vi "K2450 Set Volt.vi"(8 "error in (no error)":errorcluster {"code" format="%.0x"}, 10 "Voltage 2450":dbl, 11 "VISA resource name":refnum<visa-resource-name>) -> (0 "error out":errorcluster {"code" format="%.0x"}, 2 "Write ∆ Time [ms]":dbl format="%.4f", 3 "dup VISA Session":refnum<visa-resource-name>)   [LabVIEW 2025]
doc: "Author: Scott Hannahs <sth@magnet.fsu.edu>\n\nThis software is licensed for use under the “MIT License\"\nCopyright (c) 2025 Scott Hannahs, sth@sth@magnet.sthnet.net\n\nPermission is hereby granted, free of charge, to any person obtaining a copy of this software and associated documentation files (the \"Software\"), to deal in the Software without restriction, including without limitation the rights to use, copy, modify, merge, publish, distribute, sublicense, and/or sell copies of the Software, and to permit persons to whom the Software is furnished to do so, subject to the following conditions: The above copyright notice and this permission notice shall be included in all copies or substantial portions of the Software.\n\nTHE SOFTWARE IS PROVIDED \"AS IS\", WITHOUT WARRANTY OF ANY KIND, EXPRESS OR IMPLIED, INCLUDING BUT NOT LIMITED TO THE WARRANTIES OF MERCHANTABILITY, FITNESS FOR A PARTICULAR PURPOSE AND NONINFRINGEMENT. IN NO EVENT SHALL THE AUTHORS OR COPYRIGHT HOLDERS BE LIABLE FOR ANY CLAIM, DAMAGES OR OTHER LIABILITY, WHETHER IN AN ACTION OF CONTRACT, TORT OR OTHERWISE, ARISING FROM, OUT OF OR IN CONNECTION WITH THE SOFTWARE OR THE USE OR OTHER DEALINGS IN THE SOFTWARE."
panel:
  # "Make sure unit is set to source V\nsour:func volt\nAnd turned on\nOUTPut ON"
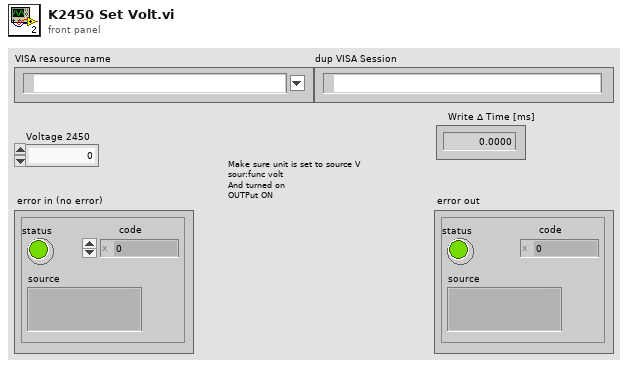
[diagram p1: front panel]
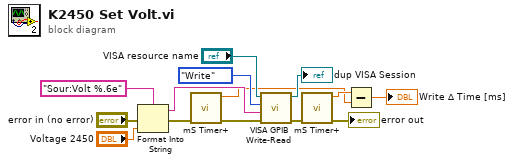
[diagram p0: block diagram]
diagram:
  n1 = Format Into String(format string="Sour:Volt %.6e" ("Command"), error in="error in (no error)", "Voltage 2450") -> (resulting string=w10:string, error out=w5:errorcluster)  [unwired: 1 in]
  n2 = call "mS Timer+.vi"("Error In"=w5) -> ("Error Out"=w4:errorcluster, "MilliSecond Timer Value"=w2:dbl)  [unwired: 9 in]
  n3 = call "VISA GPIB Write-Read.vi"("error in (no error)"=w4, "Command"=w10, "Action"=enum16{"Write", "Read", "Write & Read"}."Write", "VISA resource name"="VISA resource name") -> ("error out"=w7:errorcluster, "dup VISA Session"=→"dup VISA Session":refnum<visa-resource-name>)  [unwired: 4 in, 2 out]
  n4 = call "mS Timer+.vi"("Error In"=w7) -> ("Error Out"=→"error out":errorcluster, "MilliSecond Timer Value"=w3:dbl)  [unwired: 9 in]
  n5 = Subtract(x=w3, y=w2) -> (x-y=→"Write ∆ Time [ms]":dbl)
